vi "Query Multi Eval Meas List ACLR NR Carrier Frequency Limit Check Results.vi"(6 "Carrier Frequency (Positive)":i32(ring)=1 items=["Negative", "Positive"], 8 "error in (no error)":errorcluster, 9 "Result Type (Current)":i32(ring) items=["Current", "Average"], 10 "Instance (1)":T1=1, 11 "VISA resource name":refnum<visa-resource-name>) -> (0 "error out":errorcluster, 1 "Limit Check Results":i32[](array[numeric]), 2 "Reliability":i32, 3 "VISA resource name out":refnum<visa-resource-name>)   [LabVIEW 2020, in "Rohde&Schwarz CMWXP NR FR1 Measurement.lvlib"]
doc: "Return the ACLR limit check results for the first adjacent NR channel above (Positive) or below (Negative) the carrier frequency for all measured list mode segments.\n\nAttributes:\nRSCMWXPNRFR1M_ATTR_QUERY_MULTI_EVAL_MEAS_LIST_ACLR_NR_NEGATIVE_CURRENT_LIMIT_CHECK_RESULTS\nRSCMWXPNRFR1M_ATTR_QUERY_MULTI_EVAL_MEAS_LIST_ACLR_NR_NEGATIVE_AVERAGE_LIMIT_CHECK_RESULTS\nRSCMWXPNRFR1M_ATTR_QUERY_MULTI_EVAL_MEAS_LIST_ACLR_NR_POSITIVE_CURRENT_LIMIT_CHECK_RESULTS\nRSCMWXPNRFR1M_ATTR_QUERY_MULTI_EVAL_MEAS_LIST_ACLR_NR_POSITIVE_AVERAGE_LIMIT_CHECK_RESULTS\n\nRemote-control commands:\nCALCulate:NRSub:MEAS<i>:MEValuation:LIST:ACLR:NR:NEGativ:CURRent?\nCALCulate:NRSub:MEAS<i>:MEValuation:LIST:ACLR:NR:NEGativ:AVERage?\nCALCulate:NRSub:MEAS<i>:MEValuation:LIST:ACLR:NR:POSitiv:CURRent?\nCALCulate:NRSub:MEAS<i>:MEValuation:LIST:ACLR:NR:POSitiv:AVERage?"
uses:
  <instrlib>/Rohde&Schwarz CMWXP NR FR1 Measurement/Rohde&Schwarz CMWXP NR FR1 Measurement.lvlib
  <instrlib>/Rohde&Schwarz CMWXP NR FR1 Measurement/Private/_Instance.ctl
  <instrlib>/Rohde&Schwarz CMWXP NR FR1 Measurement/Private/rsidr_core.llb/rsidr_core.lvlib
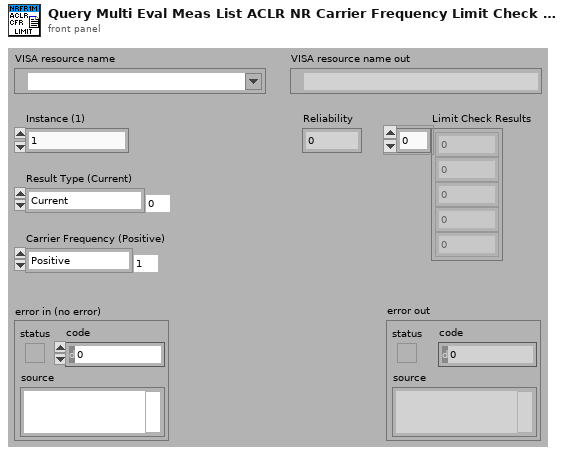
[diagram p1: front panel]
types:
  T1 = typedef "Rohde&Schwarz CMWXP NR FR1 Measurement.lvlib/_Instance.ctl" = i32
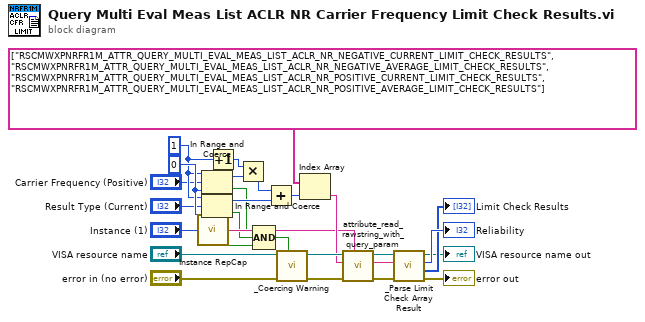
[diagram p0: block diagram]
diagram:
  w10 = 1
  w12 = 0
  n1 = call <instrlib>:"Instance RepCap.vi"("Instance In"="Instance (1)") -> ("In Range?"=w4:bool, "RepCap Identifier Out"=w24:string)  [unwired: 1 in]
  n2 = In Range and Coerce(upper limit=w10, x="Carrier Frequency (Positive)", lower limit=w12) -> (coerced(x)=w11:i32, In Range?=w2:bool)
  n3 = In Range and Coerce(upper limit=w10, x="Result Type (Current)", lower limit=w12) -> (coerced(x)=w13:i32, In Range?=w3:bool)
  n4 = Increment(x=w10) -> (x+1=w9:i32)
  n5 = Multiply(x=w9, y=w11) -> (x*y=w8:i32)
  n6 = Compound Arithmetic op=AND(w2, w3, w4) -> (w5:bool)
  n7 = Add(x=w8, y=w13) -> (x+y=w1:i32)
  n8 = call <instrlib>:"_Coercing Warning.vi"("In Range?"=w5, "error in (no error)"="error in (no error)", "VISA resource name"="VISA resource name") -> ("error out"=w25:errorcluster, "VISA resource name out"=w27:refnum<visa-resource-name>)  [unwired: 7 in]
  n9 = Index Array(array=string[] ["RSCMWXPNRFR1M_ATTR_QUERY_MULTI_EVAL_MEAS_LIST_ACLR_NR_NEGATIVE_CURRENT_LIMIT_CHECK_RESULTS", "RSCMWXPNRFR1M_ATTR_QUERY_MULTI_EVAL_MEAS_LIST_ACLR_NR_NEGATIVE_AVERAGE_LIMIT_CHECK_RESULTS", "RSCMWXPNRFR1M_ATTR_QUERY_MULTI_EVAL_MEAS_LIST_ACLR_NR_POSITIVE_CURRENT_LIMIT_CHECK_RESULTS", "RSCMWXPNRFR1M_ATTR_QUERY_MULTI_EVAL_MEAS_LIST_ACLR_NR_POSITIVE_AVERAGE_LIMIT_CHECK_RESULTS"], index=w1) -> (element=w26:string)
  n10 = call <instrlib>:"attribute_read_rawstring_with_query_param.vi"("Repeated Capability"=w24, "error in"=w25, "Attribute ID"=w26, "VISA resource name"=w27) -> ("error out"=w23:errorcluster, "Raw String out"=w22:string, "VISA resource name out"=w21:refnum<visa-resource-name>)  [unwired: 5 in]
  n11 = call <instrlib>:"_Parse Limit Check Array Result.vi"("error in (no error)"=w23, "Input String"=w22, "VISA resource name"=w21) -> ("error out"=→"error out":errorcluster, "Results"=→"Limit Check Results":i32[], "Reliability"=→"Reliability":i32, "VISA resource name out"=→"VISA resource name out":refnum<visa-resource-name>)  [unwired: 3 in, 1 out]
